vi "R(H)_VaryT_Runner.vi"() -> ()   [LabVIEW 2019]
uses:
  Components/Global 2.vi
  Components/DeltaRamp_globals.vi
  Components/B_Globals.vi
panel:
  out "Settle Progress":u8(slide) scale=0.0..100.0
  in  "Settle [Min]":dbl=1.0
  out "This Run":path=path "C:/User Data/hlb54/210227/Test_T=1p60K.txt"
  out "Last Saved":path=path "C:/User Data/hlb54/210227/Test_T=1p00K.txt"
  in  "Sample ID/Save Name":string="39A"
  in  "Save Directory":path=path "C:/User Data/hlb54/210227"
  out "dT/dt SetP":dbl
  in  "Temp Rate [K/min]":dbl=0.1
  in  "Measure":bool
  out "dH/dt SetP":dbl=0.05
  out "Field SetP":dbl=-0.5
  out "Temp SetP":dbl=1.6
  in  "Field [T] and Rate [T/min]":dbl[][](array[numeric])=[[0.5, 0.1], [-0.5, 0.05], [-1.0, 0.1], [-0.5, 0.1], [0.5, 0.05], [1.0, 0.1]]
  in  "Temps [K]":dbl[](array[numeric])=[7.3]
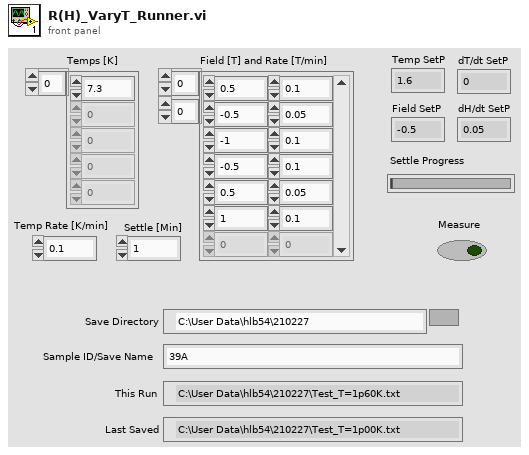
[diagram p1: front panel]
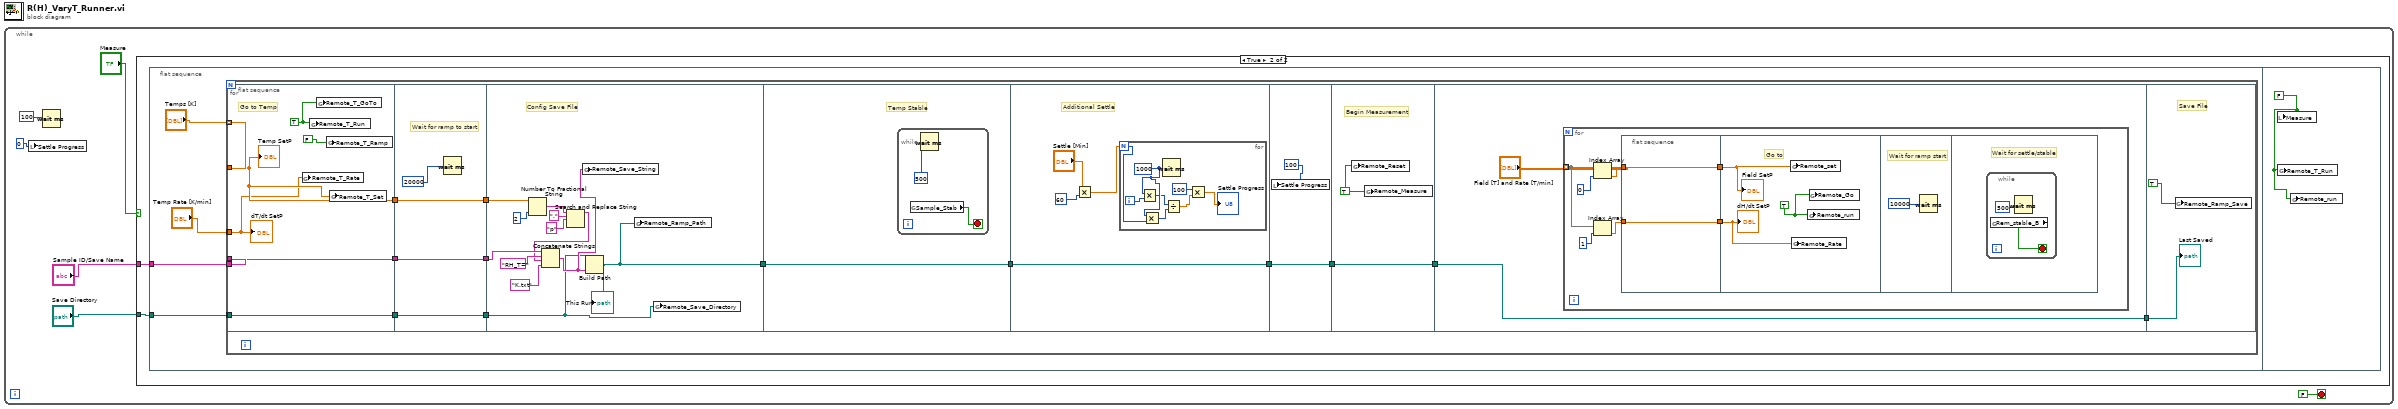
[diagram p0: block diagram]
diagram:
  n1 = while {
    stop <- FALSE stop-if-true
    n2 = local write "Settle Progress"(0) -> ()
    n3 = Wait (ms)(milliseconds to wait=100) -> ()  [unwired: 1 out]
    n4 = case shown="True" "Measure" {
      tunnel: "Sample ID/Save Name" -> [_ w8]
      tunnel: "Save Directory" -> [_ w7]
      frame False {
      }
      frame True {
        n5 = flat-sequence {
          tunnel: w8 -> [w10]
          tunnel: w7 -> [w9]
          frame #0 {
            n6 = for {
              tunnel: "Temps [K]" -> [w28] mode=indexing
              tunnel: "Temp Rate [K/min]" -> [w27]
              tunnel: w10 -> [w26]
              tunnel: w9 -> [w25]
              n7 = flat-sequence {
                tunnel: w28 -> [w30]
                tunnel: w27 -> [w29]
                tunnel: [w34] -> w18
                tunnel: w26 -> [w34]
                tunnel: w25 -> [w33]
                tunnel: [w33] -> w16
                tunnel: [w30] -> w14
                tunnel: w18 -> [w38]
                tunnel: [w38] -> w17
                tunnel: w16 -> [w37]
                tunnel: [w37] -> w15
                tunnel: w14 -> [w36]
                tunnel: [w36] -> w13
                tunnel: w17 -> [w50]
                tunnel: w15 -> [w40]
                tunnel: w13 -> [w46]
                tunnel: [w39] -> w21
                tunnel: [w51] -> w23
                tunnel: w21 -> [w51]
                tunnel: w23 -> [w57]
                tunnel: [w57] -> w22
                tunnel: w22 -> [w67]
                tunnel: [w67] -> w20
                tunnel: w20 -> [w69]
                tunnel: [w69] -> w19
                tunnel: [w70] -> w24
                tunnel: w19 -> [w70]
                tunnel: w24 -> [w88]
                frame #0 {
                  w32 = TRUE
                  # "Go to Temp"
                  n8 = global write "Global 2.vi" "Remote_T_Rate"(w29) -> ()
                  n9 = global write "Global 2.vi" "Remote_T_Run"(w32) -> ()
                  n10 = global write "Global 2.vi" "Remote_T_GoTo"(w32) -> ()
                  n11 = global write "Global 2.vi" "Remote_T_Ramp"(FALSE) -> ()
                  n12 = global write "Global 2.vi" "Remote_T_Set"(w30) -> ()
                  "Temp SetP" <- w30
                  "dT/dt SetP" <- w29
                }
                frame #1 {
                  # "Wait for ramp to start"
                  n13 = Wait (ms)(milliseconds to wait=20000) -> ()  [unwired: 1 out]
                }
                frame #2 {
                  # "Config Save File"
                  n14 = Number To Fractional String(number=w46, precision (6)=i16 2) -> (F-format string=w43:string)  [unwired: 2 in]
                  n15 = Search and Replace String(input string=w43, search string=".", replace string="p") -> (result string=w42:string)  [unwired: 5 in, 3 out]
                  n16 = Concatenate Strings(w50, "RH_T=", w42, "K.txt") -> (w41:string)
                  n17 = global write "DeltaRamp_globals.vi" "Remote_Save_String"(w41) -> ()
                  n18 = Build Path(base path=w40, name or relative path=w41) -> (appended path=w39:path)
                  "This Run" <- w39
                  n19 = global write "DeltaRamp_globals.vi" "Remote_Ramp_Path"(w39) -> ()
                  n20 = global write "DeltaRamp_globals.vi" "Remote_Save_Directory"(w40) -> ()
                }
                frame #3 {
                  # "Temp Stable"
                  n21 = while {
                    stop <- w53 stop-if-true
                    n22 = global read "Global 2.vi" "Sample_Stab"() -> (w53:bool)
                    n23 = Wait (ms)(milliseconds to wait=500) -> ()  [unwired: 1 out]
                  }
                }
                frame #4 {
                  # "Additional Settle"
                  n24 = Multiply(x="Settle [Min]", y=60) -> (x*y=w54:dbl)
                  n25 = for {
                    N: w54 -> [w64]
                    i -> [w65]
                    w63 = 1000
                    n26 = Multiply(x=w63, y=w65) -> (x*y=w61:i32)
                    n27 = Multiply(x=w63, y=w64) -> (x*y=w62:i32)
                    n28 = Wait (ms)(milliseconds to wait=w63) -> ()  [unwired: 1 out]
                    n29 = Divide(x=w61, y=w62) -> (x/y=w59:dbl)
                    n30 = Multiply(x=100, y=w59) -> (x*y=→"Settle Progress":dbl)
                  }
                }
                frame #5 {
                  n31 = local write "Settle Progress"(100) -> ()
                }
                frame #6 {
                  w68 = TRUE
                  # "Begin Measurement"
                  n32 = global write "DeltaRamp_globals.vi" "Remote_Reset"(w68) -> ()
                  n33 = global write "DeltaRamp_globals.vi" "Remote_Measure"(w68) -> ()
                }
                frame #7 {
                  n34 = for {
                    tunnel: "Field [T] and Rate [T/min]" -> [w76] mode=indexing
                    n35 = Index Array(array=w76, index=1) -> (element=w74:dbl)
                    n36 = Index Array(array=w76, index=0) -> (element=w77:dbl)
                    n37 = flat-sequence {
                      tunnel: w74 -> [w79]
                      tunnel: w77 -> [w80]
                      tunnel: [w80] -> w73
                      tunnel: [w79] -> w72
                      tunnel: w73 -> [w82]
                      tunnel: w72 -> [w81]
                      frame #0 {
                      }
                      frame #1 {
                        w83 = TRUE
                        # "Go to"
                        n38 = global write "B_Globals.vi" "Remote_set"(w82) -> ()
                        n39 = global write "B_Globals.vi" "Remote_Rate"(w81) -> ()
                        n40 = global write "B_Globals.vi" "Remote_run"(w83) -> ()
                        n41 = global write "B_Globals.vi" "Remote_Go"(w83) -> ()
                        "Field SetP" <- w82
                        "dH/dt SetP" <- w81
                      }
                      frame #2 {
                        # "Wait for ramp start"
                        n42 = Wait (ms)(milliseconds to wait=10000) -> ()  [unwired: 1 out]
                      }
                      frame #3 {
                        # "Wait for settle/stable"
                        n43 = while {
                          stop <- w85 stop-if-true
                          n44 = global read "B_Globals.vi" "Rem_stable_B"() -> (w85:bool)
                          n45 = Wait (ms)(milliseconds to wait=500) -> ()  [unwired: 1 out]
                        }
                      }
                    }
                  }
                }
                frame #8 {
                  # "Save File"
                  n46 = global write "DeltaRamp_globals.vi" "Remote_Ramp_Save"(TRUE) -> ()
                  "Last Saved" <- w88
                }
              }
            }
          }
          frame #1 {
            w89 = FALSE
            n47 = local write "Measure"(w89) -> ()
            n48 = global write "Global 2.vi" "Remote_T_Run"(w89) -> ()
            n49 = global write "B_Globals.vi" "Remote_run"(w89) -> ()
          }
        }
      }
    }
  }
